vi "Read Device Type.vi"(8 "error in (no error)":errorcluster, 10 "node":u8, 11 "ProPar in":refnum<class "PL Bronkhorst ProPar.lvclass">) -> (0 "error out":errorcluster, 2 "device type":string, 3 "ProPar out":refnum<class "PL Bronkhorst ProPar.lvclass">)   [LabVIEW 2015, in "PL Bronkhorst ProPar.lvclass"]
doc: "Reads device type of the specified <b>node</b>."
uses:
  PL Bronkhorst ProPar.lvclass
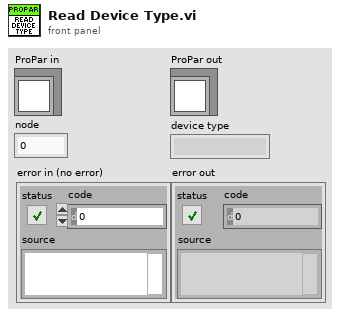
[diagram p1: front panel]
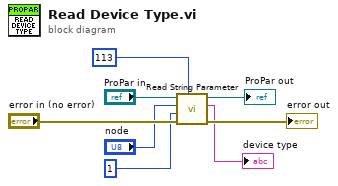
[diagram p0: block diagram]
diagram:
  n1 = call "Read String Parameter.vi"("process number"=u8 113, "error in (no error)"="error in (no error)", "parameter number"=u8 1 ("process number"), "node"="node", "ProPar in"="ProPar in") -> ("error out"=→"error out":errorcluster, "value"=→"device type":string, "ProPar out"=→"ProPar out":refnum<class "PL Bronkhorst ProPar.lvclass">)  [unwired: 4 in]
